vi "Bat+sound+recovery+solution.vi"() -> ()   [LabVIEW 2011]
uses:
  <vilib>/sound2/lvsound2.llb/Sound File Read Open.vi
  <vilib>/sound2/lvsound2.llb/Sound File Read (DBL).vi
panel:
  in  "Path":path
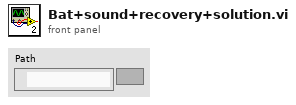
[diagram p1: front panel]
types:
  T1 = typedef "Sound File Refnum.ctl" = refnum<file>
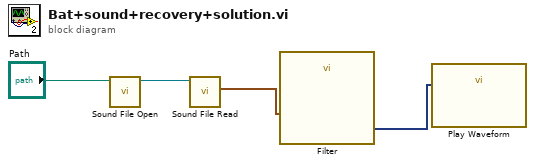
[diagram p0: block diagram]
diagram:
  n1 = call-poly <vilib>:"Sound File Open.vi"("path"="Path") -> ("sound file refnum"=w3:T1)  [unwired: 9 in, 1 out]
  n2 = call-poly <vilib>:"Sound File Read.vi"("sound file refnum"=w3) -> ("data"=w2:waveform(dbl)[])  [unwired: 6 in, 4 out]
  n3 = call "Filter"("Signal"=w2) -> ("Filtered Signal"=w1:dynamicdata)  [unwired: 9 in, 1 out]
  n4 = call "Play Waveform"("Data"=w1) -> ()  [unwired: 18 in, 1 out]
